vi "XML-Write.vi"(8 "error in (no error)":errorcluster, 10 "Data":variant, 11 "XML File Path":path) -> (0 "error out":errorcluster, 2 "XML String":string, 3 "XML File Path(duplicate)":path)   [LabVIEW 2024]
uses:
  <vilib>/Utility/xml.llb/Write to XML File(string).vi
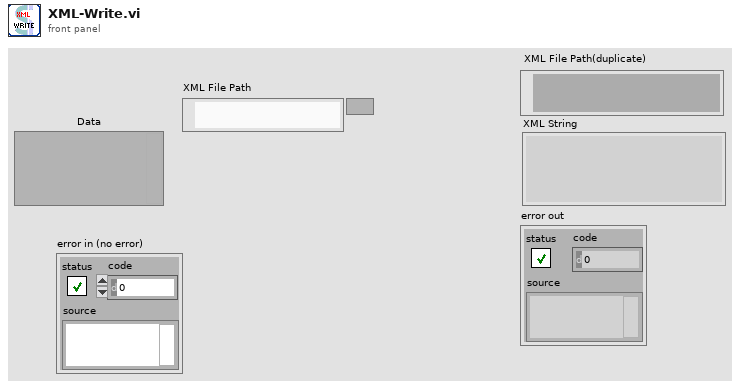
[diagram p1: front panel]
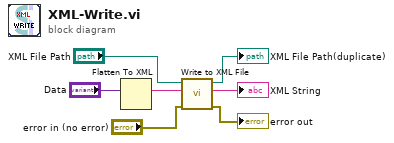
[diagram p0: block diagram]
diagram:
  n1 = Flatten To XML(6:"Data") -> (2:w7:string)
  n2 = call-poly <vilib>:"Write to XML File.vi"("error in (no error)"="error in (no error)", "XML Input"=w7, "XML File Path"="XML File Path") -> ("error out"=→"error out":errorcluster, "XML String"=→"XML String":string, "XML File Path(duplicate)"=→"XML File Path(duplicate)":path)  [unwired: 6 in]
